vi "Base Test.vi"(5 "Invert?":bool, 7 "Additional Data":variant, 10 "y":dbl, 11 "x":dbl) -> (2 "Equal?":bool)   [LabVIEW 2018]
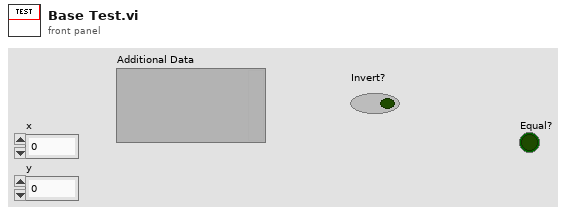
[diagram p1: front panel]
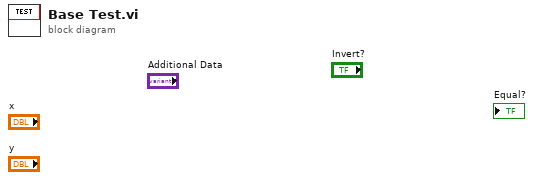
[diagram p0: block diagram]
diagram:
